vi "obj_ClientSrv Client Access State.vi"(0 "method (ensure)":T2, 7 "access level (observer)":T1, 11 "error in (no error)":errorcluster) -> (8 "certificate":string, 15 "error out":errorcluster)   [LabVIEW 2012]
doc: "Client-side object that manages the server access state. The {ensure} method will try to return or acquire a certificate of the appropriate access level. A certificate of the appropriate access level is required when performing a remote call on server-side VIs. This VI should therefore be placed on the diagram before the \"Call By Reference\" node. Since certificates are prone to change over time, do not wire the output of this VI through a loop boundary so as to ensure an as-fresh-as-possible certificate.\n\nIf operator access is required, and no corresponding certificate is held yet or when the held certificate is no longer tests as being valid on the server, a password will be queried by popping up a dialog that explains the reason for the failed access (no certificate yet, other client holding certificate, certicate timed out, etc.). If a previously aquired certificate is still valid, the method returns without an error.\n\nThe {release} method releases the currently held operator certificate so as to secure the running client and/or signal other clients that it is safe to acquire operator access."
uses:
  typedefs/t_ClientSrv Client Access State Methods.ctl
  typedefs/t_ClientSrv Access Levels.ctl
  typedefs/t_ClientSrv Server Access Methods.ctl
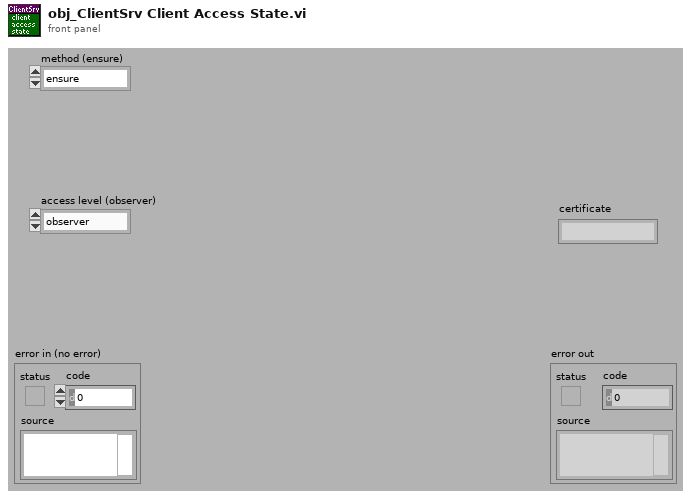
[diagram p1: front panel]
types:
  T1 = typedef "t_ClientSrv Access Levels.ctl" = enum16{"observer", "operator", "local"}
  T2 = typedef "t_ClientSrv Client Access State Methods.ctl" = enum16{"ensure", "release"}
  T3 = typedef "t_ClientSrv Server Access Methods.ctl" = enum16{"validate access", "test access", "release access", "get name"}
  T4 = typedef "ClientSrv Server Access_srv.ctl" = refnum<vi>
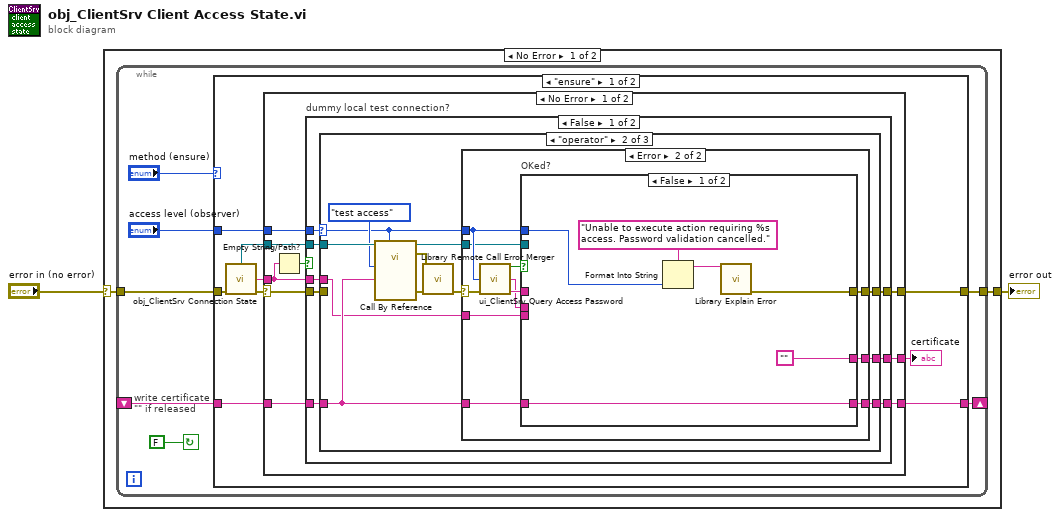
[diagram p0: block diagram]
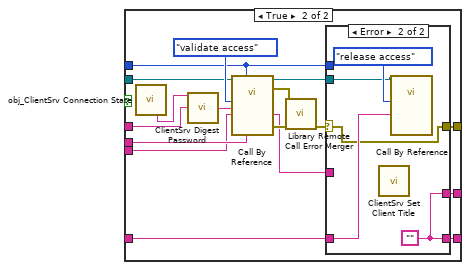
[diagram p4: hidden frame]
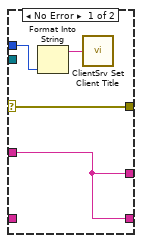
[diagram p5: hidden frame]
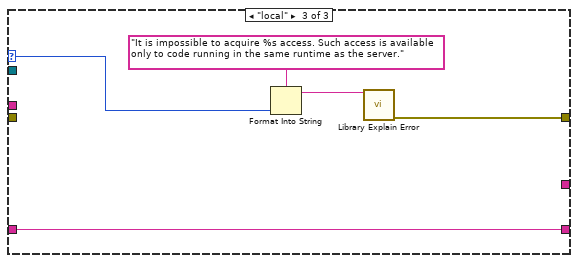
[diagram p6: hidden frame]
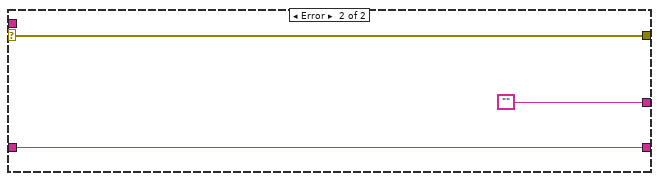
[diagram p8: hidden frame]
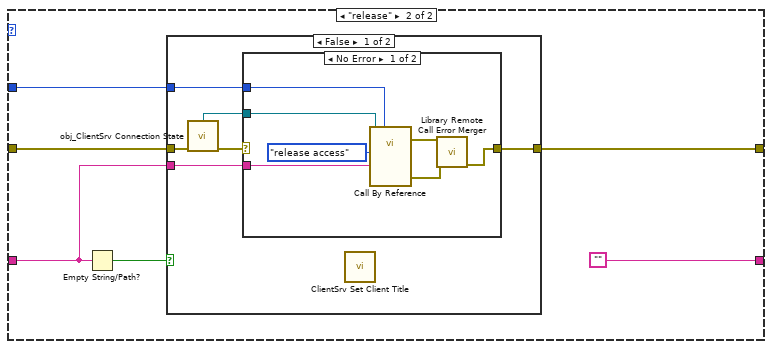
[diagram p9: hidden frame]
diagram:
  n1 = case shown="No Error" "error in (no error)" {
    selector: "error in (no error)" -> [w4 w130]
    tunnel: [w3 w130] -> w1
    frame No Error {
      n2 = while {
        tunnel: w4 -> [w11]
        tunnel: [w10] -> w3
        shift-right: [w6] -> _
        shift-left: _ -> [w9]
        stop <- FALSE continue-if-true
        # "write certificate\n\"\" if released"
        n3 = case shown="\"ensure\"" "method (ensure)" {
          tunnel: w11 -> [w15 w111]
          tunnel: [w20 w113] -> w10
          tunnel: w9 -> [w18 w110]
          tunnel: [w17 ""] -> w6
          tunnel: "access level (observer)" -> [w19 w112]
          frame "ensure" {
            n4 = call "obj_ClientSrv Connection State.vi"("error in (no error)"=w15) -> ("server access"=w12:T4, "observer certificate"=w13:string, "error out"=w16:errorcluster)  [unwired: 7 in, 5 out]
            n5 = case shown="No Error" w16 {
              selector: w16 -> [w23 w108]
              tunnel: w12 -> [w29 _]
              tunnel: [w26 w108] -> w20
              tunnel: w19 -> [w24 _]
              tunnel: w18 -> [w28 w107]
              tunnel: [w27 w107] -> w17
              tunnel: [w25 ""] -> w14
              tunnel: w13 -> [w22 _]
              frame No Error {
                n6 = Empty String/Path?(string/path=w22) -> (empty?=w21:bool)
                n7 = case "dummy local test connection?" shown="False" w21 {
                  tunnel: w29 -> [w37 _]
                  tunnel: w28 -> [w36 w103]
                  tunnel: [w35 w103] -> w27
                  tunnel: [w34 w105] -> w26
                  tunnel: [w33 w104] -> w25
                  tunnel: w24 -> [w32 _]
                  tunnel: w22 -> [w31 w104]
                  tunnel: w23 -> [w30 w105]
                  frame False {
                    n8 = case shown="\"operator\"" w32 {
                      selector: w32 -> [_ w42 w100]
                      tunnel: w37 -> [_ w52 _]
                      tunnel: w36 -> [w39 w47 w102]
                      tunnel: [w39 w46 w102] -> w35
                      tunnel: [w38 w45 w101] -> w34
                      tunnel: [w40 w43 _] -> w33
                      tunnel: w31 -> [w40 w41 _]
                      tunnel: w30 -> [w38 _ _]
                      frame "observer" {
                      }
                      frame "operator" {
                        n9 = call-by-ref "?"(reference=w52, "method"=t_ClientSrv_Server_Access_Methods."test access", "access level"=w42, "certificate in"=w47) -> (reference out=w44:T4, error out=w51:errorcluster, 15:"error out"=w50:errorcluster)  [unwired: 11 in, 2 out]
                        n10 = call "Library Remote Call Error Merger.vi"("call by reference node error"=w51, "called VI error (no error)"=w50) -> ("error out"=w48:errorcluster)  [unwired: 13 in]
                        n11 = case shown="Error" w48 {
                          selector: w48 -> [w54 w65]
                          tunnel: w47 -> [w53 w63]
                          tunnel: w42 -> [_ w60]
                          tunnel: [w53 w62] -> w46
                          tunnel: [w54 w61] -> w45
                          tunnel: w44 -> [_ w59]
                          tunnel: [w53 w58] -> w43
                          tunnel: w41 -> [_ w55]
                          frame No Error {
                          }
                          frame Error {
                            n12 = call "ui_ClientSrv Query Access Password.vi"("access level"=w60, "test error in"=w65) -> ("OKed?"=w64:bool, "access reason out"=w56:string, "access password out"=w57:string)  [unwired: 11 in]
                            n13 = case "OKed?" shown="False" w64 {
                              tunnel: w63 -> [w71 w80]
                              tunnel: [w71 w82] -> w62
                              tunnel: [w70 w78] -> w61
                              tunnel: w60 -> [w69 w83]
                              tunnel: w59 -> [_ w85]
                              tunnel: ["" w77] -> w58
                              tunnel: w57 -> [_ w72]
                              tunnel: w56 -> [_ w76]
                              tunnel: w55 -> [_ w75]
                              frame False {
                                n14 = Format Into String(format string="Unable to execute action requiring %s access. Password validation cancelled.", w69) -> (resulting string=w68:string)  [unwired: 2 in, 1 out]
                                n15 = call "Library Explain Error.vi"("explanation prefix (none)"=w68) -> ("explained error"=w70:errorcluster)  [unwired: 14 in]
                              }
                              frame True {
                                n16 = call "obj_ClientSrv Connection State.vi"() -> ("server"=w73:string)  [unwired: 8 in, 7 out]
                                n17 = call "ClientSrv Digest Password.vi"("server name (none)"=w73, "password"=w72) -> ("SHA-1 digest"=w74:string)  [unwired: 13 in]
                                n18 = call-by-ref "?"(reference=w85, "method"=t_ClientSrv_Server_Access_Methods."validate access", "access level"=w83, "digest"=w74, "certificate in"=w75, "access reason"=w76) -> (reference out=w79:T4, error out=w86:errorcluster, "certificate/name out"=w81:string, 15:"error out"=w87:errorcluster)  [unwired: 9 in, 1 out]
                                n19 = call "Library Remote Call Error Merger.vi"("call by reference node error"=w86, "called VI error (no error)"=w87) -> ("error out"=w84:errorcluster)  [unwired: 13 in]
                                n20 = case shown="Error" w84 {
                                selector: w84 -> [w90 w94]
                                tunnel: w83 -> [w92 _]
                                tunnel: [w89 w93] -> w82
                                tunnel: w81 -> [w89 _]
                                tunnel: w80 -> [_ w96]
                                tunnel: w79 -> [_ w95]
                                tunnel: [w90 w94] -> w78
                                tunnel: [w89 w93] -> w77
                                frame No Error {
                                n21 = Format Into String(w92) -> (resulting string=w91:string)  [unwired: 3 in, 1 out]
                                n22 = call "ClientSrv Set Client Title.vi"("write access (none)"=w91) -> ()  [unwired: 15 in]
                                }
                                frame Error {
                                w93 = ""
                                n23 = call "ClientSrv Set Client Title.vi"() -> ()  [unwired: 16 in]
                                n24 = call-by-ref "?"(reference=w95, "method"=t_ClientSrv_Server_Access_Methods."release access", "certificate in"=w96) -> ()  [unwired: 12 in, 5 out]
                                }
                                }
                              }
                            }
                          }
                        }
                      }
                      frame "local" {
                        n25 = Format Into String(format string="It is impossible to acquire %s access. Such access is available only to code running in the same runtime as the server.", w100) -> (resulting string=w99:string)  [unwired: 2 in, 1 out]
                        n26 = call "Library Explain Error.vi"("explanation prefix (none)"=w99) -> ("explained error"=w101:errorcluster)  [unwired: 14 in]
                      }
                    }
                  }
                  frame True {
                  }
                }
              }
              frame Error {
              }
            }
            "certificate" <- w14
          }
          frame "release" {
            n27 = Empty String/Path?(string/path=w110) -> (empty?=w109:bool)
            n28 = case shown="False" w109 {
              tunnel: [w119 w129] -> w113
              tunnel: w110 -> [w118 _]
              tunnel: w112 -> [w117 _]
              tunnel: w111 -> [w116 w129]
              frame False {
                n29 = call "obj_ClientSrv Connection State.vi"("error in (no error)"=w116) -> ("server access"=w115:T4, "error out"=w120:errorcluster)  [unwired: 7 in, 6 out]
                n30 = case shown="No Error" w120 {
                  selector: w120 -> [_ w128]
                  tunnel: w115 -> [w127 _]
                  tunnel: [w121 w128] -> w119
                  tunnel: w118 -> [w123 _]
                  tunnel: w117 -> [w122 _]
                  frame No Error {
                    n31 = call-by-ref "?"(reference=w127, "method"=t_ClientSrv_Server_Access_Methods."release access", "access level"=w122, "certificate in"=w123) -> (error out=w126:errorcluster, 15:"error out"=w125:errorcluster)  [unwired: 11 in, 3 out]
                    n32 = call "Library Remote Call Error Merger.vi"("call by reference node error"=w126, "called VI error (no error)"=w125) -> ("error out"=w121:errorcluster)  [unwired: 13 in]
                  }
                  frame Error {
                  }
                }
                n33 = call "ClientSrv Set Client Title.vi"() -> ()  [unwired: 16 in]
              }
              frame True {
              }
            }
          }
        }
      }
    }
    frame Error {
    }
  }
  "error out" <- w1
